vi "Make Protection Signal.vi"(11 "Node Ptr":T1=18446744073709551615 format="%.0x") -> ()   [LabVIEW 2015, in "Protection and Rolling Counter Addon System Explorer.lvlib"]
uses:
  Protection and Rolling Counter Addon System Explorer.lvlib
  <vilib>/NI Veristand/Custom Device API/Custom Device Item Ref.ctl
  <vilib>/NI Veristand/Custom Device API/Custom Device Channel Type.ctl
  Shared/SubVIs/GUID Lookup.vi
  <vilib>/NI Veristand/Custom Device API/Custom Device API.lvlib
  Shared/Protection and Rolling Counter Addon Shared.lvlib
  <vilib>/NI Veristand/Custom Device Tools/Custom Device Utility Library/Custom Device Utility Library.lvlib
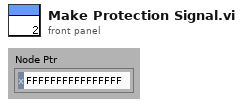
[diagram p1: front panel]
types:
  T1 = typedef "Custom Device API.lvlib/Custom Device Item Ref.ctl" = u64
  T2 = typedef "Custom Device API.lvlib/Custom Device Channel Type.ctl" = enum16{"Input", "Output"}
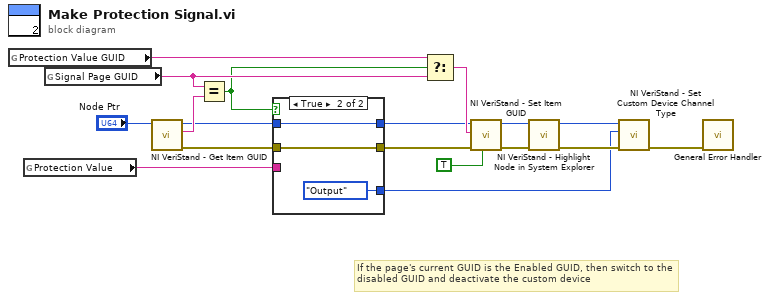
[diagram p0: block diagram]
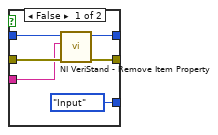
[diagram p2: hidden frame]
diagram:
  # "If the page's current GUID is the Enabled GUID, then switch to the disabled GUID and deactivate the custom device"
  n1 = global read "GUID Lookup.vi" "Protection Value GUID"() -> (w13:string)
  n2 = global read "GUID Lookup.vi" "Protection Value"() -> (w6:string)
  n3 = global read "GUID Lookup.vi" "Signal Page GUID"() -> (w14:string)
  n4 = call <vilib>:"NI VeriStand - Get Item GUID.vi"("Item Ref in"="Node Ptr") -> ("error out"=w10:errorcluster, "GUID"=w17:string, "Item Ref out"=w8:T1)  [unwired: 8 in]
  n5 = Equal?(x=w14, y=w17) -> (x = y?=w5:bool)
  n6 = case shown="True" w5 {
    tunnel: w10 -> [w24 w26]
    tunnel: [w23 w26] -> w9
    tunnel: w8 -> [w22 w27]
    tunnel: [w21 w27] -> w7
    tunnel: w6 -> [w20 _]
    tunnel: [Custom_Device_Channel_Type."Input" ("Type") Custom_Device_Channel_Type."Output" ("Type")] -> w1
    frame False {
      n7 = call <vilib>:"NI VeriStand - Remove Item Property.vi"("error in (no error)"=w24, "Property Name"=w20, "Item Ref in"=w22) -> ("error out"=w23:errorcluster, "Item Ref out"=w21:T1)  [unwired: 6 in, 1 out]
    }
    frame True {
    }
  }
  n8 = Select(t=w13, s=w5, f=w14) -> (s? t:f=w15:string)
  n9 = call <vilib>:"NI VeriStand - Set Item GUID.vi"("Refresh System Explorer Tree? (F)"=TRUE, "error in (no error)"=w9, "GUID"=w15, "Item Ref in"=w7) -> ("error out"=w11:errorcluster, "Item Ref out"=w12:T1)  [unwired: 6 in]
  n10 = call <vilib>:"NI VeriStand - Highlight Node in System Explorer.vi"("error in (no error)"=w11, "Item Ref in"=w12) -> ("error out"=w3:errorcluster, "Node Ptr dup"=w4:T1)  [unwired: 8 in]
  n11 = call <vilib>:"NI VeriStand - Set Custom Device Channel Type.vi"("error in (no error)"=w3, "Type"=w1, "Channel Ref in"=w4) -> ("error out"=w2:errorcluster)  [unwired: 7 in, 1 out]
  n12 = call <vilib>:"General Error Handler.vi"("error in (no error)"=w2) -> ()  [unwired: 10 in, 5 out]
